vi "Actor Core.vi"(8 "error in":errorcluster, 11 "CS++GoBangClient in":refnum<class "CS++GoBangClient.lvclass">) -> (0 "error out":errorcluster, 3 "Actor out":refnum<class "Actor.lvclass">)   [LabVIEW 2014, in "GoBang.lvlib" / "CS++GoBangClient.lvclass"]
doc: "(<B>Filename</B>: Actor Framework.lvlib:Actor.lvclass:Actor Core.vi)\n\nReceives messages to the actor, reacts to them, and initiates any error handling that may shut the actor down.\n\nDescendant classes may override this VI to append parallel tasks for the actor to complete while it handles messages. Overrides use the Call Parent Method node."
uses:
  CS++GoBangClient.lvclass
  <vilib>/ActorFramework/Actor/Actor.lvclass
  typdefs/BoardField.ctl
  typdefs/GameState.ctl
  <vilib>/NI/Actors/Linked Network Actor/Linked Network Actor/Linked Network Actor.lvclass
  CS++GoBangClient.lvclass/CS++GoBangClient.ctl
  CS++GoBangServer Messages/Analyse Board Msg/Analyse Board Msg.lvclass
  CS++GoBangServer Messages/Analyse Board Msg/Analyse Board Msg.lvclass/Analyse Board Msg.ctl
  CS++GoBangServer Messages/JoinGame Msg/JoinGame Msg.lvclass
  CS++GoBangServer Messages/JoinGame Msg/JoinGame Msg.lvclass/JoinGame Msg.ctl
  <vilib>/ActorFramework/Actor/Actor.lvclass/Actor.ctl
  <vilib>/ActorFramework/Message Enqueuer/Message Enqueuer.lvclass/Message Enqueuer.ctl
  <vilib>/ActorFramework/Message Enqueuer/Init from Existing Queue.vi
  <vilib>/ActorFramework/Message Enqueuer/Enqueue.vi
  <vilib>/ActorFramework/Message Priority Queue/Priority Enqueue.vi
  <vilib>/ActorFramework/Message Enqueuer/Message Enqueuer.lvclass
  <vilib>/ActorFramework/Stop Msg/Stop Msg.lvclass
  GoBang.lvlib
  <vilib>/NI/Actors/Linked Network Actor/Linked Network Actor Messages/Connect Msg/Connect Msg.lvclass
  <vilib>/NI/Actors/Linked Network Actor/Linked Network Actor Messages/Disconnect Msg/Disconnect Msg.lvclass
  <vilib>/NI/Actors/Linked Network Actor/Linked Network Actor Messages/Transmit Network Message Msg/Transmit Network Message Msg.lvclass
panel:
  in  "Connect":bool
  in  "OppColor":T1
  out "Opponnents name":string
  in  "Color":T1
  in  "Your name":string
  in  "stone":T1
  in  "stop":bool
  in  "State":T2
  out "GameBoard":T1[][](array[typedef])
  out "White won":bool
  out "Black won":bool
  out "Game over":bool
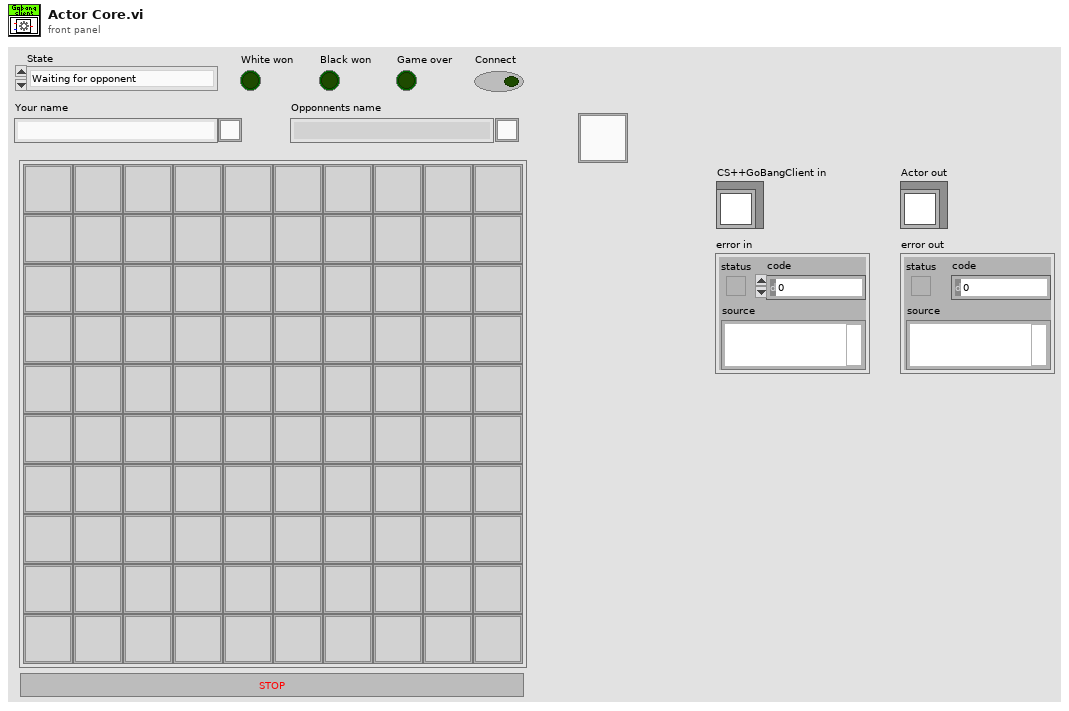
[diagram p1: front panel]
types:
  T1 = typedef "GoBang.lvlib/BoardField.ctl" = u8
  T2 = typedef "GoBang.lvlib/GameState.ctl" = enum16{"Waiting for opponent", "White to move", "Black to move", "Game over, white won", "Game over, black won"}
  T3 = typedef "LVPositionTypeDef.ctl" = cluster{"Left":i32, "Top":i32}
  T4 = typedef "LVBoundsTypeDef.ctl" = cluster{"Width":u32, "Height":u32}
  T5 = enum32{"Invalid", "Standard", "Closed", "Hidden", "Minimized", "Maximized"}
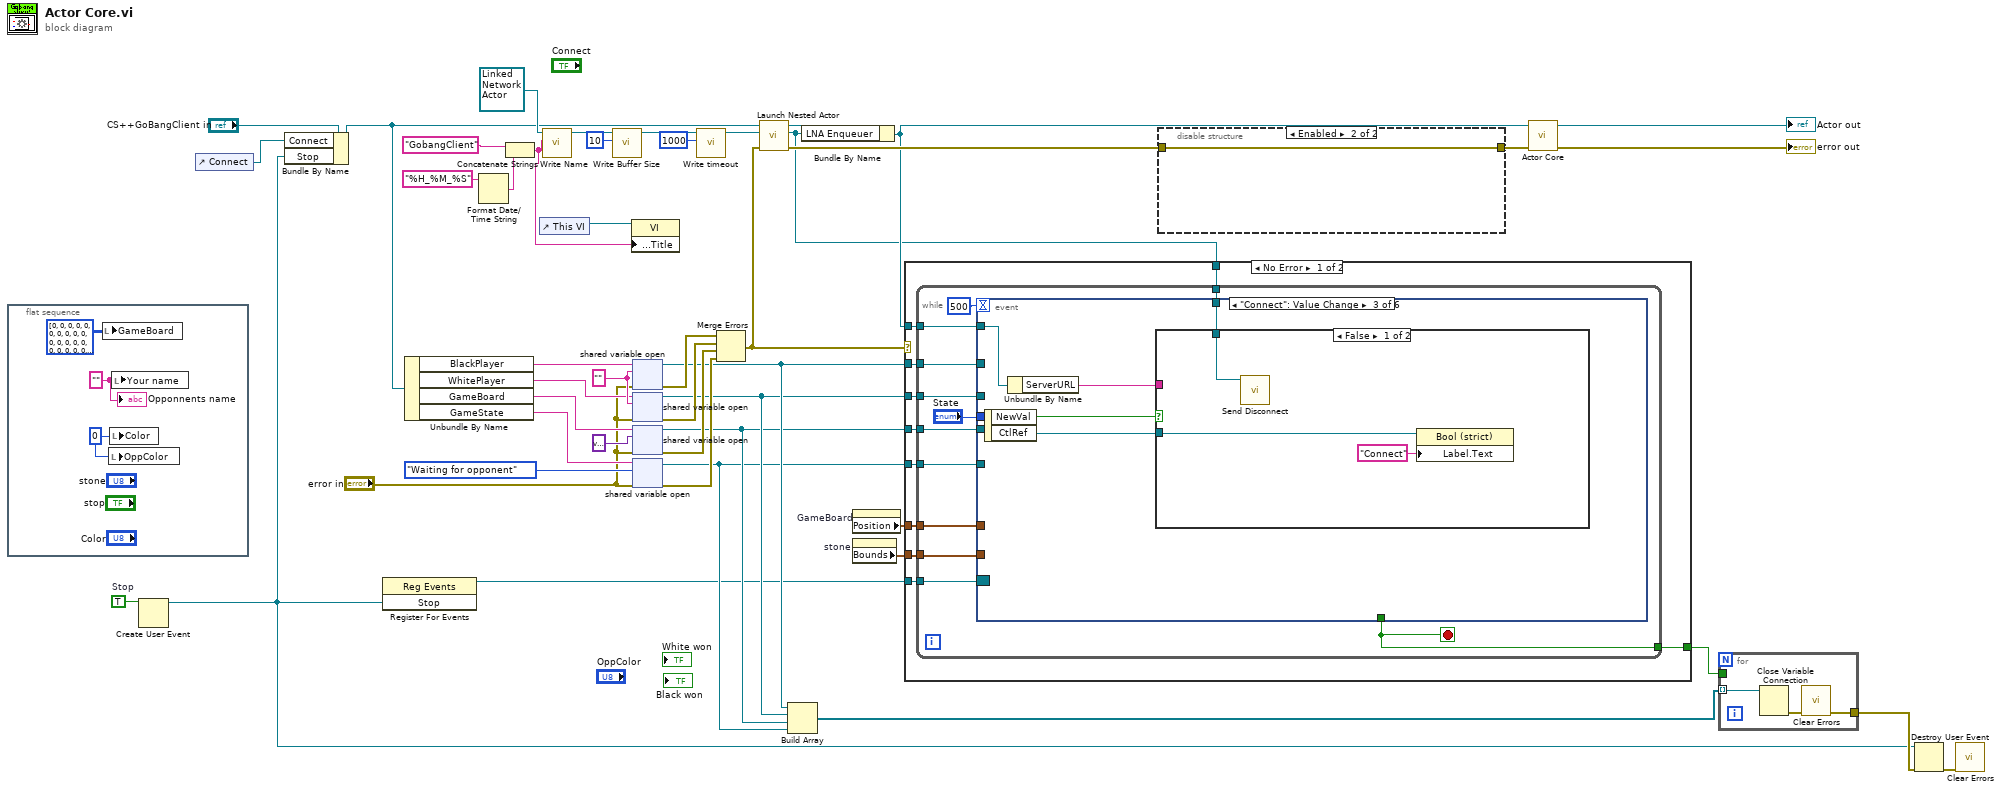
[diagram p0: block diagram]
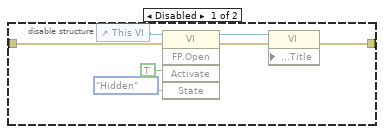
[diagram p2: hidden frame]
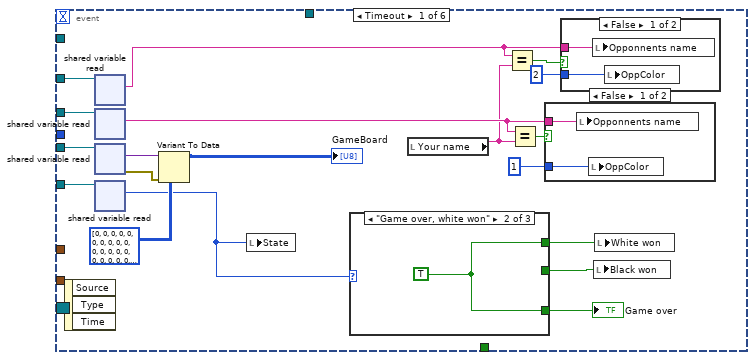
[diagram p3: hidden frame]
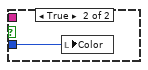
[diagram p4: hidden frame]
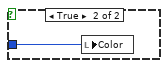
[diagram p5: hidden frame]
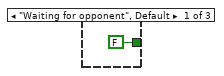
[diagram p6: hidden frame]
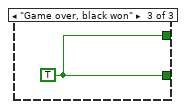
[diagram p7: hidden frame]
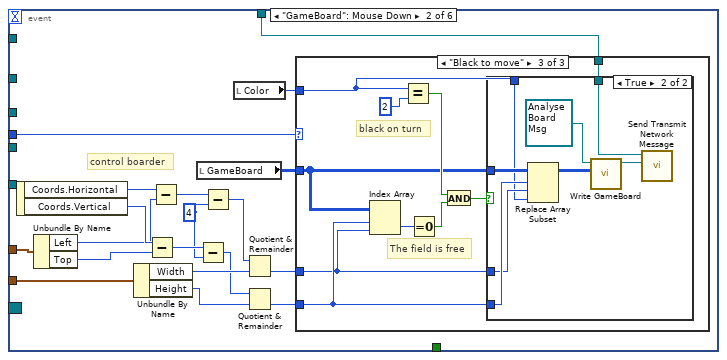
[diagram p8: hidden frame]
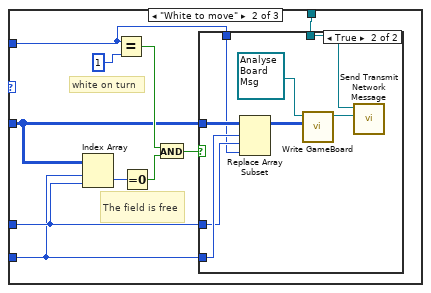
[diagram p10: hidden frame]
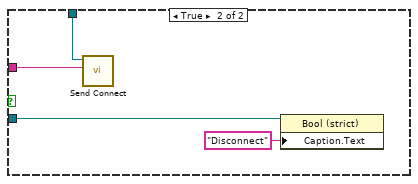
[diagram p13: hidden frame]
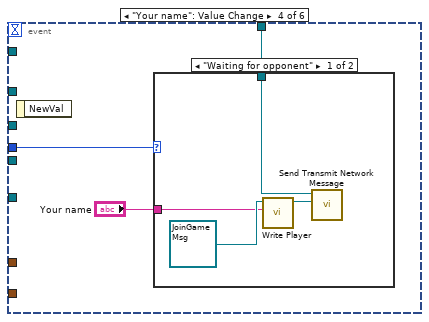
[diagram p14: hidden frame]
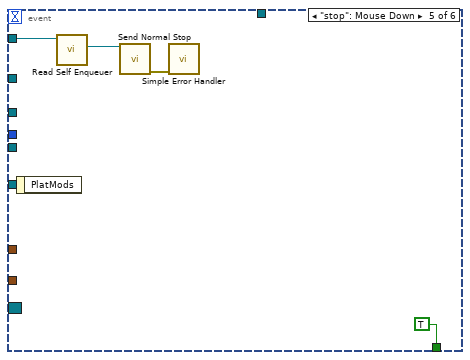
[diagram p16: hidden frame]
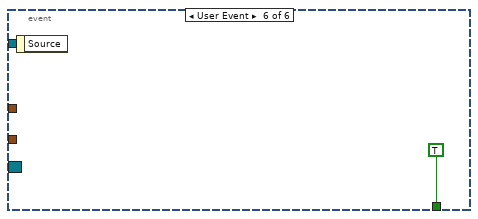
[diagram p17: hidden frame]
diagram:
  w14 = TRUE  # Stop
  w43 = ""
  n1 = flat-sequence {
    frame #0 {
      w49 = T1 0 ("Color")
      w48 = "" ("Your name")
      n2 = local write "GameBoard"(T1[][] [[0, 0, 0, 0, 0, 0, 0, 0, 0, 0], [0, 0, 0, 0, 0, 0, 0, 0, 0, 0], [0, 0, 0, 0, 0, 0, 0, 0, 0, 0], [0, 0, 0, 0, 0, 0, 0, 0, 0, 0], [0, 0, 0, 0, 0, 0, 0, 0, 0, 0], [0, 0, 0, 0, 0, 0, 0, 0, 0, 0], [0, 0, 0, 0, 0, 0, 0, 0, 0, 0], [0, 0, 0, 0, 0, 0, 0, 0, 0, 0], [0, 0, 0, 0, 0, 0, 0, 0, 0, 0], [0, 0, 0, 0, 0, 0, 0, 0, 0, 0]] ("GameBoard")) -> ()
      n3 = local write "OppColor"(w49) -> ()
      n4 = local write "Color"(w49) -> ()
      n5 = local write "Your name"(w48) -> ()
      "Opponnents name" <- w48
    }
  }
  n6 = Create User Event(user event datatype=w14) -> (user event=w4:refnum<user-event>)  [unwired: 1 in, 1 out]
  n7 = control-ref of="Connect"() -> (w3:refnum<vi>)
  n8 = Bundle By Name(cluster="CS++GoBangClient in", "Connect"=w3, "Stop"=w4) -> (w11:refnum<class "CS++GoBangClient.lvclass">)
  n9 = register-events(w4) -> (reference out=w10:refnum<event-registration>)  [unwired: 2 in, 1 out]
  n10 = Unbundle By Name(w11) -> ("BlackPlayer"=w44:string, "WhitePlayer"=w42:string, "GameBoard"=w41:string, "GameState"=w40:string)
  n11 = Format Date/Time String(time format string (%c)="%H_%M_%S") -> (date/time string=w6:string)  [unwired: 2 in]
  n12 = Concatenate Strings("GobangClient" ("Name"), w6) -> (w1:string)
  n13 = control-ref of="This VI"() -> (w2:refnum<vi>)
  n14 = call <vilib>:"Write Name.vi"("Name"=w1, "Network Actor in"=refnum<class "Linked Network Actor.lvclass"> refnum ("Network Actor.lvlib:Network Actor.lvclass")) -> ("Network Actor out"=w27:refnum<class "Linked Network Actor.lvclass">)  [unwired: 9 in]
  n15 = call <vilib>:"Write Buffer Size.vi"("Buffer Size"=10, "Network Actor in"=w27) -> ("Network Actor out"=w28:refnum<class "Linked Network Actor.lvclass">)  [unwired: 9 in]
  n16 = property class="VI"(reference=w2, "Front Panel.Title"=w1) -> ()  [unwired: 1 in, 2 out]
  n17 = shared-variable-open(w44, "error in", w43) -> (w22:refnum<k21>, w37:errorcluster)  [unwired: 1 in]
  n18 = shared-variable-open(w42, "error in", w43) -> (w21:refnum<k21>, w36:errorcluster)  [unwired: 1 in]
  n19 = shared-variable-open(w41, "error in", variant) -> (w20:refnum<k21>, w35:errorcluster)  [unwired: 1 in]
  n20 = shared-variable-open(w40, "error in", GameState."Waiting for opponent" ("State")) -> (w19:refnum<k21>, w34:errorcluster)  [unwired: 1 in]
  n21 = call <vilib>:"Write timeout.vi"("timeout"=1000, "Network Actor in"=w28) -> ("Network Actor out"=w25:refnum<class "Linked Network Actor.lvclass">)  [unwired: 9 in]
  n22 = Merge Errors(w37, w36, w35, w34) -> (w24:errorcluster)
  n23 = call <vilib>:"Launch Nested Actor.vi"("error in (no error)"=w24, "Nested Actor"=w25, "Caller Actor in"=w11) -> ("error out"=w23:errorcluster, "Nested Actor's Enqueuer"=w12:refnum<class "Message Enqueuer.lvclass">, "Caller Actor out"=w15:refnum<class "CS++GoBangClient.lvclass">)  [unwired: 6 in]
  n24 = Build Array(w22, w21, w20, w19) -> (w18:refnum<k21>[])
  n25 = Bundle By Name(cluster=w15, "LNA Enqueuer"=w12) -> (w13:refnum<class "CS++GoBangClient.lvclass">)
  n26 = property on="GameBoard" class="Arr (strict)"() -> ("Position"=w45:T3)  [unwired: 2 in, 2 out]
  n27 = property on="stone" class="Ring (strict)"() -> ("Bounds"=w46:T4)  [unwired: 2 in, 2 out]
  n28 = case shown="No Error" w24 {
    tunnel: w46 -> [w60 _]
    tunnel: w45 -> [w59 _]
    tunnel: w22 -> [w58 _]
    tunnel: w21 -> [w57 _]
    tunnel: w20 -> [w56 _]
    tunnel: w19 -> [w55 _]
    tunnel: w12 -> [w54 _]
    tunnel: [w53 _] -> w17
    tunnel: w13 -> [w52 _]
    tunnel: w10 -> [w51 _]
    frame No Error {
      n29 = while {
        tunnel: w60 -> [w72]
        tunnel: w59 -> [w71]
        tunnel: w54 -> [w69]
        tunnel: w58 -> [w67]
        tunnel: w57 -> [w66]
        tunnel: w56 -> [w65]
        tunnel: w55 -> [w64]
        tunnel: [w63] -> w53
        tunnel: w52 -> [w62]
        tunnel: w51 -> [w61]
        stop <- w63 stop-if-true
        n30 = event shown="[2] \"Connect\": Value Change" {
          selector: w61 -> [_ _ _ _ _ _]
          dyn-events: _ -> [_ _ _ _ _ _]
          timeout: 500 -> [_ _ _ _ _ _]
          tunnel: [_ _ _ _ TRUE TRUE] -> w63
          tunnel: w72 -> [_ w119 _ _ _ _]
          tunnel: w71 -> [_ w114 _ _ _ _]
          tunnel: "State" -> [_ w104 _ w170 _ _]
          tunnel: w69 -> [_ w101 w160 w168 _ _]
          tunnel: w67 -> [w91 _ _ _ _ _]
          tunnel: w66 -> [w90 _ _ _ _ _]
          tunnel: w65 -> [w89 _ _ _ _ _]
          tunnel: w64 -> [w88 _ _ _ _ _]
          tunnel: w62 -> [_ _ w159 _ w175 _]
          event Timeout {
            n31 = event-data() -> ()  [unwired: 1 in, 3 out]
            n32 = shared-variable-read(w91) -> (w73:string)  [unwired: 1 in, 3 out]
            n33 = shared-variable-read(w90) -> (w77:string)  [unwired: 1 in, 3 out]
            n34 = shared-variable-read(w89) -> (w85:errorcluster, w87:variant)  [unwired: 1 in, 2 out]
            n35 = shared-variable-read(w88) -> (w80:T2)  [unwired: 1 in, 3 out]
            n36 = Variant To Data(error in=w85, type=T1[][] [[0, 0, 0, 0, 0, 0, 0, 0, 0, 0], [0, 0, 0, 0, 0, 0, 0, 0, 0, 0], [0, 0, 0, 0, 0, 0, 0, 0, 0, 0], [0, 0, 0, 0, 0, 0, 0, 0, 0, 0], [0, 0, 0, 0, 0, 0, 0, 0, 0, 0], [0, 0, 0, 0, 0, 0, 0, 0, 0, 0], [0, 0, 0, 0, 0, 0, 0, 0, 0, 0], [0, 0, 0, 0, 0, 0, 0, 0, 0, 0], [0, 0, 0, 0, 0, 0, 0, 0, 0, 0], [0, 0, 0, 0, 0, 0, 0, 0, 0, 0]] ("GameBoard"), Variant=w87) -> (data=→"GameBoard":T1[][])  [unwired: 1 out]
            n37 = local write "State"(w80) -> ()
            n38 = case shown="\"Game over, white won\"" w80 {
              tunnel: [FALSE ("White won") w99 w100] -> w83
              tunnel: [_ _ w100] -> w82
              tunnel: [_ w99 _] -> w81
              frame "Waiting for opponent", Default {
              }
              frame "Game over, white won" {
                w99 = TRUE ("White won")
              }
              frame "Game over, black won" {
                w100 = TRUE ("White won")
              }
            }
            "Game over" <- w83
            n39 = local read "Your name"() -> (w74:string)
            n40 = Equal?(x=w73, y=w74) -> (x = y?=w76:bool)
            n41 = Equal?(x=w77, y=w74) -> (x = y?=w79:bool)
            n42 = case shown="False" w79 {
              tunnel: w77 -> [w96 _]
              tunnel: T1 1 ("Color") -> [w95 w97]
              frame False {
                n43 = local write "Opponnents name"(w96) -> ()
                n44 = local write "OppColor"(w95) -> ()
              }
              frame True {
                n45 = local write "Color"(w97) -> ()
              }
            }
            n46 = case shown="False" w76 {
              tunnel: w73 -> [w93 _]
              tunnel: T1 2 ("Color") -> [w92 w94]
              frame False {
                n47 = local write "Opponnents name"(w93) -> ()
                n48 = local write "OppColor"(w92) -> ()
              }
              frame True {
                n49 = local write "Color"(w94) -> ()
              }
            }
            n50 = local write "Black won"(w82) -> ()
            n51 = local write "White won"(w81) -> ()
          }
          event "GameBoard": Mouse Down {
            w107 = 4 ("y 2")
            # "control boarder"
            n52 = event-data() -> ("Coords.Horizontal"=w118:i32, "Coords.Vertical"=w116:i32)  [unwired: 1 in]
            n53 = Unbundle By Name(w114) -> ("Left"=w113:i32, "Top"=w112:i32)
            n54 = Unbundle By Name(w119) -> ("Width"=w117:u32, "Height"=w115:u32)
            n55 = Subtract(x=w116, y=w112) -> (x-y=w110:i32)
            n56 = Subtract(x=w118, y=w113) -> (x-y=w111:i32)
            n57 = local read "GameBoard"() -> (w103:T1[][])
            n58 = Subtract(x=w110, y=w107) -> (x-y=w108:i32)
            n59 = Subtract(x=w111, y=w107) -> (x-y=w109:i32)
            n60 = local read "Color"() -> (w102:T1)
            n61 = Quotient & Remainder(x=w109, y=w117) -> (floor(x/y)=w106:u32)  [unwired: 1 out]
            n62 = Quotient & Remainder(x=w108, y=w115) -> (floor(x/y)=w105:u32)  [unwired: 1 out]
            n63 = case shown="\"Black to move\"" w104 {
              tunnel: w106 -> [_ w122 w146]
              tunnel: w105 -> [_ w121 w147]
              tunnel: w103 -> [_ w124 w141]
              tunnel: w102 -> [_ w120 w139]
              tunnel: w101 -> [_ w125 w138]
              frame "Waiting for opponent", Default {
              }
              frame "White to move" {
                # "white on turn"
                # "The field is free"
                n64 = Index Array(array=w124, index (row)=w121, index (col)=w122) -> (element=w129:T1)
                n65 = Equal?(x=w120, y=T1 1) -> (x = y?=w127:bool)
                n66 = Equal To 0?(x=w129) -> (x = 0?=w128:bool)
                n67 = And(x=w127, y=w128) -> (x .and. y?=w123:bool)
                n68 = case shown="True" w123 {
                  tunnel: w121 -> [_ w137]
                  tunnel: w122 -> [_ w136]
                  tunnel: w124 -> [_ w135]
                  tunnel: w120 -> [_ w134]
                  tunnel: w125 -> [_ w130]
                  frame False {
                  }
                  frame True {
                    n69 = Replace Array Subset(array=w135, new element=w134, index (row)=w137, index (col)=w136) -> (w132:T1[][])
                    n70 = call "Write GameBoard.vi"("GameBoard"=w132, "Analyse Board Msg in"=refnum<class "Analyse Board Msg.lvclass"> refnum ("GoBang.lvlib:Analyse Board Msg.lvclass")) -> ("Analyse Board Msg out"=w133:refnum<class "Analyse Board Msg.lvclass">)  [unwired: 9 in]
                    n71 = call <vilib>:"Send Transmit Network Message.vi"("Message"=w133, "Message Enqueuer"=w130) -> ()  [unwired: 8 in, 2 out]
                  }
                }
              }
              frame "Black to move" {
                # "black on turn"
                # "The field is free"
                n72 = Index Array(array=w141, index (row)=w147, index (col)=w146) -> (element=w145:T1)
                n73 = Equal?(x=w139, y=T1 2) -> (x = y?=w142:bool)
                n74 = Equal To 0?(x=w145) -> (x = 0?=w143:bool)
                n75 = And(x=w142, y=w143) -> (x .and. y?=w144:bool)
                n76 = case shown="True" w144 {
                  tunnel: w147 -> [_ w155]
                  tunnel: w146 -> [_ w154]
                  tunnel: w141 -> [_ w153]
                  tunnel: w139 -> [_ w152]
                  tunnel: w138 -> [_ w151]
                  frame False {
                  }
                  frame True {
                    n77 = Replace Array Subset(array=w153, new element=w152, index (row)=w155, index (col)=w154) -> (w150:T1[][])
                    n78 = call "Write GameBoard.vi"("GameBoard"=w150, "Analyse Board Msg in"=refnum<class "Analyse Board Msg.lvclass"> refnum ("GoBang.lvlib:Analyse Board Msg.lvclass")) -> ("Analyse Board Msg out"=w148:refnum<class "Analyse Board Msg.lvclass">)  [unwired: 9 in]
                    n79 = call <vilib>:"Send Transmit Network Message.vi"("Message"=w148, "Message Enqueuer"=w151) -> ()  [unwired: 8 in, 2 out]
                  }
                }
              }
            }
          }
          event "Connect": Value Change {
            n80 = event-data() -> ("NewVal"=w157:bool, "CtlRef"=w156:refnum<vi>)  [unwired: 1 in]
            n81 = Unbundle By Name(w159) -> ("ServerURL"=w158:string)
            n82 = case shown="False" w157 {
              tunnel: w160 -> [w163 w167]
              tunnel: w158 -> [_ w166]
              tunnel: w156 -> [w162 w165]
              frame False {
                n83 = call <vilib>:"Send Disconnect.vi"("Message Enqueuer"=w163) -> ()  [unwired: 9 in, 2 out]
                n84 = property class="Bool (strict)"(reference=w162, "Label.Text"="Connect") -> ()  [unwired: 1 in, 2 out]
              }
              frame True {
                n85 = call <vilib>:"Send Connect.vi"("URL"=w166, "Message Enqueuer"=w167) -> ()  [unwired: 8 in, 2 out]
                n86 = property class="Bool (strict)"(reference=w165, "Caption.Text"="Disconnect" ("Label.Text")) -> ()  [unwired: 1 in, 2 out]
              }
            }
          }
          event "Your name": Value Change {
            n87 = event-data() -> ()  [unwired: 1 in, 1 out]
            n88 = case shown="\"Waiting for opponent\"" w170 {
              tunnel: "Your name" -> [w172 _]
              tunnel: w168 -> [w174 _]
              frame "Waiting for opponent" {
                n89 = call "Write Player.vi"("Player"=w172, "JoinGame Msg in"=refnum<class "JoinGame Msg.lvclass"> refnum ("GoBang.lvlib:JoinGame Msg.lvclass")) -> ("JoinGame Msg out"=w171:refnum<class "JoinGame Msg.lvclass">)  [unwired: 9 in]
                n90 = call <vilib>:"Send Transmit Network Message.vi"("Message"=w171, "Message Enqueuer"=w174) -> ()  [unwired: 8 in, 2 out]
              }
              frame "White to move", Default {
              }
            }
          }
          event "stop": Mouse Down {
            n91 = event-data() -> ()  [unwired: 1 in, 1 out]
            n92 = call <vilib>:"Read Self Enqueuer.vi"("Actor"=w175) -> ("Self Enqueuer"=w176:refnum<class "Message Enqueuer.lvclass">)  [unwired: 10 in]
            n93 = call <vilib>:"Send Normal Stop.vi"("Message Enqueuer"=w176) -> ("error out"=w177:errorcluster)  [unwired: 10 in]
            n94 = call <vilib>:"Simple Error Handler.vi"("error in (no error)"=w177) -> ()  [unwired: 4 in, 5 out]
          }
          event User Event {
            n95 = event-data() -> ()  [unwired: 1 in, 1 out]
          }
        }
      }
    }
    frame Error {
    }
  }
  n96 = disable-structure shown="Enabled" {
    disable-tunnel: [w181 w187] -> w32
    disable-tunnel: w23 -> [w180 w187]
    frame Disabled {
      n97 = control-ref of="This VI"() -> (w184:refnum<vi>)
      n98 = invoke class="VI" method="FP.Open"(reference=w184, error in=w180, "Activate"=TRUE ("Activate?"), "State"=T5."Hidden") -> (reference out=w183:refnum<vi>, error out=w182:errorcluster)  [unwired: 1 in, 3 out]
      n99 = property class="VI" props=["Front Panel.Title"](reference=w183, error in=w182) -> (error out=w181:errorcluster)  [unwired: 1 in, 1 out]
    }
    frame Enabled {
    }
  }
  n100 = call-parent "Actor Core.vi"("error in"=w32, "Actor in"=w13) -> ("error out"=→"error out":errorcluster, "Actor out"=→"Actor out":refnum<class "Actor.lvclass">)  [unwired: 8 in]
  n101 = for {
    tunnel: w18 -> [w190] mode=indexing
    tunnel: w17 -> [_]
    tunnel: [w188] -> w8
    n102 = Close Variable Connection(11:w190) -> (0:w189:errorcluster)  [unwired: 1 in]
    n103 = call <vilib>:"Clear Errors.vi"("error in (no error)"=w189) -> ("error out"=w188:errorcluster)  [unwired: 5 in, 1 out]
  }
  n104 = Destroy User Event(user event=w4, error in=w8) -> (error out=w7:errorcluster)
  n105 = call <vilib>:"Clear Errors.vi"("error in (no error)"=w7) -> ()  [unwired: 5 in, 2 out]
